vi "HV VSet Single.vi"(8 "Voltage":string, 11 "Channel":string) -> (3 "standard output":string)   [LabVIEW 2018, in "HV QMH.lvlib"]
uses:
  HV QMH.lvlib
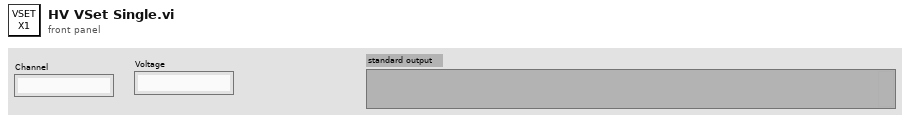
[diagram p1: front panel]
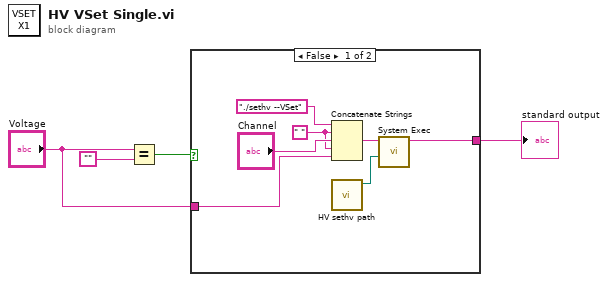
[diagram p0: block diagram]
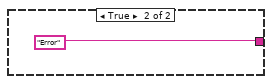
[diagram p2: hidden frame]
diagram:
  n1 = Equal?(x="Voltage", y="") -> (x = y?=w3:bool)
  n2 = case shown="False" w3 {
    tunnel: "Voltage" -> [w6 _]
    tunnel: [w5 "Error"] -> w1
    frame False {
      w7 = " " ("string")
      n3 = Concatenate Strings("./sethv --VSet" ("string"), w7, "Channel", w7, w6) -> (w9:string)
      n4 = call "HV sethv path.vi"() -> ("sethv filepath"=w11:path)  [unwired: 11 in]
      n5 = call <vilib>:"System Exec.vi"("working directory"=w11, "command line"=w9) -> ("standard output"=w5:string)  [unwired: 6 in, 3 out]
    }
    frame True {
    }
  }
  "standard output" <- w1
